vi "Control Sain Board Relays (INTERNAL VOLTS ONLY).vi"(8 "error in":errorcluster, 9 "Voltage":T1=enum."+3.3V", 11 "Device Name":string) -> (0 "error out":errorcluster)   [LabVIEW 2015]
uses:
  Internal Voltages.ctl
panel:
  in  "*(type *) &x 2":string="Dev1/port2/line0,Dev1/port2/line1,Dev1/port2/line2,Dev1/port2/line3,Dev1/port2/line4,Dev1/port2/line5"
  out "*(type *) &x":tag
  out "output array (reversed)":bool[](array[boolean])
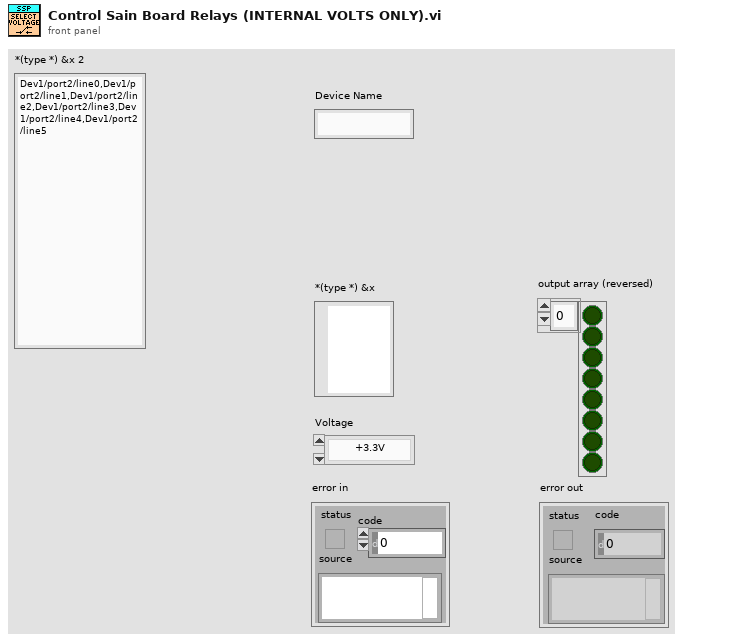
[diagram p1: front panel]
types:
  T1 = typedef "Internal Voltages.ctl" = enum16{"REF-2.5", "+3.3V", "+5.2V", "+5.2VA", "-5.2VA", "+1.6V", "NONE"}
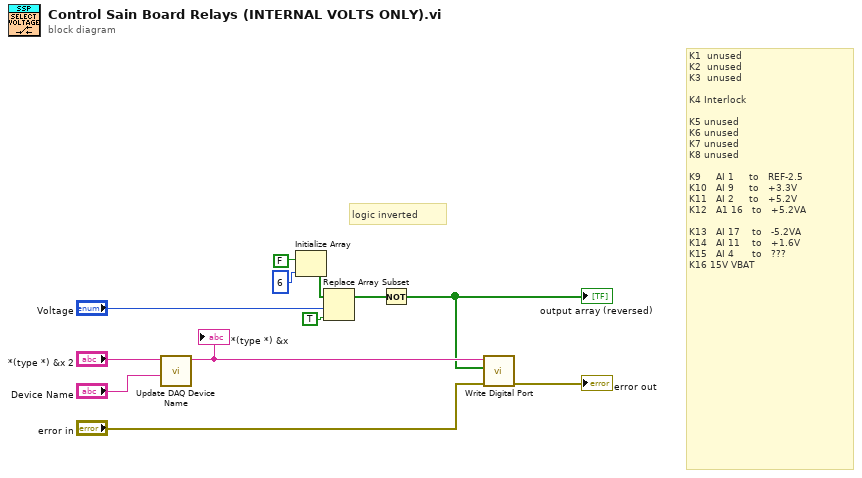
[diagram p0: block diagram]
diagram:
  # "logic inverted"
  # "K1  unused \nK2  unused\nK3  unused\n\nK4 Interlock\n\nK5 unused\nK6 unused\nK7 unused\nK8 unused\n\nK9     AI 1     to   REF-2.5\nK10   AI 9     to   +3.3V\nK11   AI 2     to   +5.2V\nK12   A1 16   to   +5.2VA\n\nK13   AI 17    to   -5.2VA\nK14   AI 11    to   +1.6V\nK15   AI 4      to   ??? \nK16 15V VBAT"
  n1 = call "Update DAQ Device Name.vi"("Device Name"="Device Name", "Lines in (String)"="*(type *) &x 2") -> ("Lines out (DAQmx Physical Channels)"=w3:tag)  [unwired: 9 in]
  "*(type *) &x" <- w3
  n2 = Initialize Array(FALSE, 6 ("dimension size")) -> (w6:bool[])
  n3 = Replace Array Subset(array=w6, new element=TRUE, index="Voltage") -> (w5:bool[])
  n4 = Not(x=w5) -> (.not. x?=w1:bool[])
  "output array (reversed)" <- w1
  n5 = call "Write Digital Port.vi"("error in"="error in", "Data"=w1, "Line(s)"=w3) -> ("error out"=→"error out":errorcluster)  [unwired: 8 in]
